vi "Gif.CreatePictureArray.vi"(1 "gloal color table":u32[](array[numeric]), 2 "GraphicControlExtension":T2, 3 "Logical Screen Description":T1, 5 "Index Array":i32[](array[numeric]), 7 "init":bool, 9 "offset":i32, 11 "error in (no error)":errorcluster, 12 "local color table":u32[](array[numeric]), 13 "ImageDescriptor":T3, 14 "bgcolor":u32) -> (4 "image out":u32[][](array[colorbox]), 10 "offset out":i32, 15 "error out":errorcluster)   [LabVIEW 2019]
uses:
  Gif.ImageDescriptor.ctl
  Gif.GraphicControlExtension.ctl
  Gif.LogicalScreenDescriptior.ctl
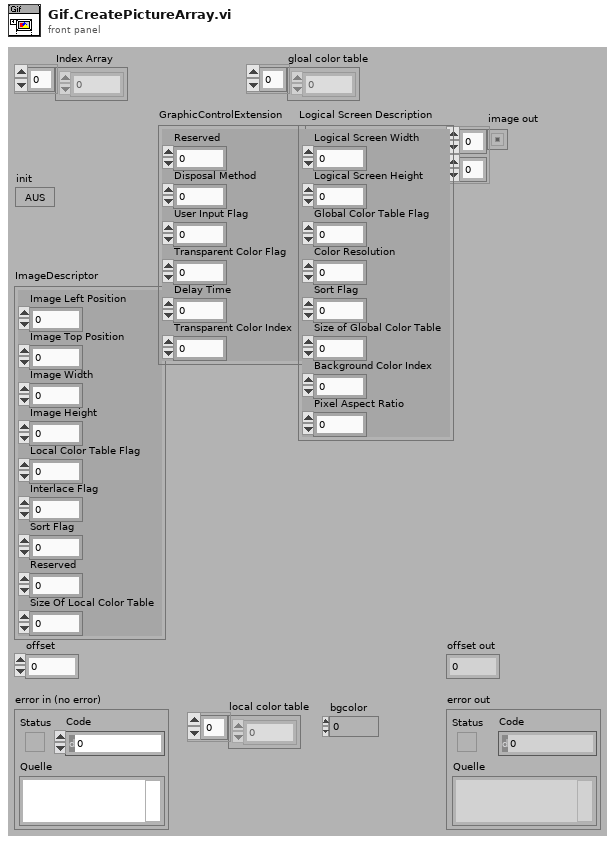
[diagram p1: front panel]
types:
  T1 = typedef "Gif.LogicalScreenDescriptior.ctl" = cluster{"Logical Screen Width":u16, "Logical Screen Height":u16, "Global Color Table Flag":u8, "Color Resolution":u8, "Sort Flag":u8, "Size of Global Color Table":u8, "Background Color Index":u8, "Pixel Aspect Ratio":u8}
  T2 = typedef "Gif.GraphicControlExtension.ctl" = cluster{"Reserved":u8, "Disposal Method":u8, "User Input Flag":u8, "Transparent Color Flag":u8, "Delay Time":u16, "Transparent Color Index":u8}
  T3 = typedef "Gif.ImageDescriptor.ctl" = cluster{"Image Left Position":u16, "Image Top Position":u16, "Image Width":u16, "Image Height":u16, "Local Color Table Flag":u8, "Interlace Flag":u8, "Sort Flag":u8, "Reserved":u8, "Size Of Local Color Table":u8}
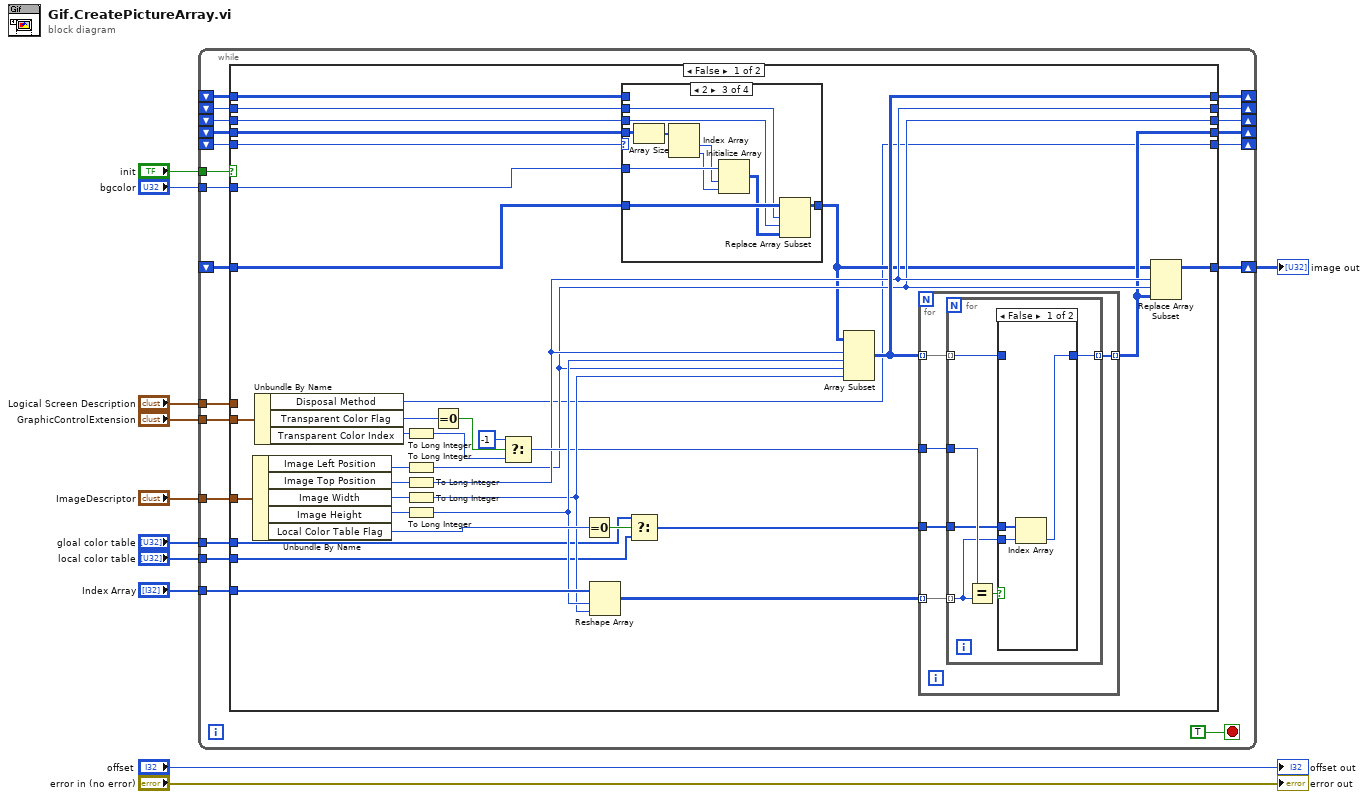
[diagram p0: block diagram]
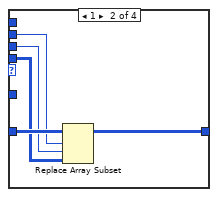
[diagram p3: hidden frame]
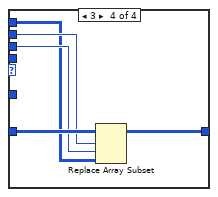
[diagram p4: hidden frame]
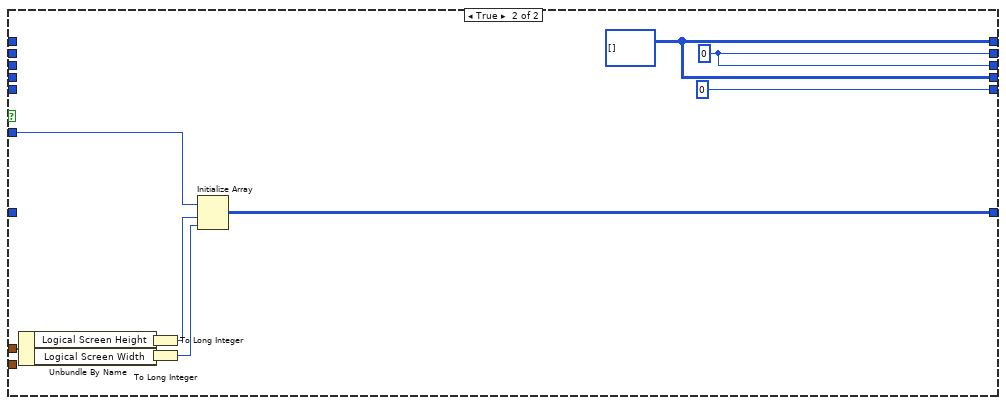
[diagram p6: hidden frame]
diagram:
  n1 = while {
    tunnel: "ImageDescriptor" -> [w32]
    tunnel: "Logical Screen Description" -> [w25]
    tunnel: "GraphicControlExtension" -> [w30]
    tunnel: "Index Array" -> [w28]
    tunnel: "local color table" -> [w27]
    tunnel: "gloal color table" -> [w14]
    shift-right: [w24] -> _
    shift-left: _ -> [w18]
    shift-right: [w23] -> _
    shift-left: _ -> [w17]
    shift-right: [w22] -> _
    shift-left: _ -> [w16]
    shift-right: [w21] -> _
    shift-left: _ -> [w15]
    shift-right: [w20] -> _
    shift-left: _ -> [w19]
    shift-right: [w31] -> w9
    shift-left: _ -> [w29]
    tunnel: "init" -> [w13]
    tunnel: "bgcolor" -> [w12]
    stop <- TRUE stop-if-true
    n2 = case shown="False" w13 {
      tunnel: w32 -> [w67 _]
      tunnel: [w64 w107] -> w31
      tunnel: w30 -> [w59 _]
      tunnel: w29 -> [w33 _]
      tunnel: w28 -> [w57 _]
      tunnel: w27 -> [w54 _]
      tunnel: w25 -> [_ w105]
      tunnel: [w47 w106] -> w24
      tunnel: [w46 w113] -> w23
      tunnel: [w45 w113] -> w22
      tunnel: [w44 w106] -> w21
      tunnel: [w42 u8 0] -> w20
      tunnel: w19 -> [w41 _]
      tunnel: w18 -> [w40 _]
      tunnel: w17 -> [w39 _]
      tunnel: w16 -> [w38 _]
      tunnel: w15 -> [w37 _]
      tunnel: w14 -> [w35 _]
      tunnel: w12 -> [w34 w108]
      frame False {
        n3 = Unbundle By Name(w67) -> ("Image Left Position"=w63:u16, "Image Top Position"=w62:u16, "Image Width"=w60:u16, "Image Height"=w61:u16, "Local Color Table Flag"=w66:u8)
        n4 = Unbundle By Name(w59) -> ("Disposal Method"=w42:u8, "Transparent Color Flag"=w52:u8, "Transparent Color Index"=w58:u8)
        n5 = To Long Integer(number=w58) -> (32bit integer=w50:i32)
        n6 = To Long Integer(number=w63) -> (32bit integer=w45:i32)
        n7 = To Long Integer(number=w62) -> (32bit integer=w46:i32)
        n8 = To Long Integer(number=w60) -> (32bit integer=w55:i32)
        n9 = To Long Integer(number=w61) -> (32bit integer=w56:i32)
        n10 = Equal To 0?(x=w52) -> (x = 0?=w51:bool)
        n11 = Select(t=-1, s=w51, f=w50) -> (s? t:f=w49:i32)
        n12 = Equal To 0?(x=w66) -> (x = 0?=w65:bool)
        n13 = Reshape Array(w57, w56, w55) -> (w53:i32[][])
        n14 = case shown="2" w41 {
          tunnel: w33 -> [w68 w73 w83 w88]
          tunnel: [w68 w72 w82 w87] -> w43
          tunnel: w40 -> [_ _ _ w84]
          tunnel: w39 -> [_ w70 w81 w86]
          tunnel: w38 -> [_ w69 w80 w85]
          tunnel: w37 -> [_ w71 w78 _]
          tunnel: w34 -> [_ _ w79 _]
          frame 0, Default {
          }
          frame 1 {
            n15 = Replace Array Subset(array=w73, new element=w71, index (row)=w70, index (col)=w69) -> (w72:u32[][])
          }
          frame 2 {
            n16 = Array Size(array=w78) -> (size(s)=w77:i32[])
            n17 = Index Array(array=w77) -> (element #1=w76:i32, element #2=w75:i32)  [unwired: 2 in]
            n18 = Initialize Array(w79, w76, w75) -> (w74:u32[][])
            n19 = Replace Array Subset(array=w83, new element=w74, index (row)=w81, index (col)=w80) -> (w82:u32[][])
          }
          frame 3 {
            n20 = Replace Array Subset(array=w88, new element=w84, index (row)=w86, index (col)=w85) -> (w87:u32[][])
          }
        }
        n21 = Select(t=w35, s=w65, f=w54) -> (s? t:f=w36:u32[])
        n22 = Array Subset(array=w43, index (row)=w46, length (row)=w56, index (col)=w45, length (col)=w55) -> (w47:u32[][])
        n23 = for {
          tunnel: w47 -> [w93] mode=indexing
          tunnel: w53 -> [w92] mode=indexing
          tunnel: w36 -> [w91]
          tunnel: w49 -> [w90]
          tunnel: [w89] -> w44 mode=indexing
          n24 = for {
            tunnel: w93 -> [w97] mode=indexing
            tunnel: w92 -> [w94] mode=indexing
            tunnel: w91 -> [w95]
            tunnel: w90 -> [w99]
            tunnel: [w96] -> w89 mode=indexing
            n25 = Equal?(x=w99, y=w94) -> (x = y?=w98:bool)
            n26 = case shown="False" w98 {
              tunnel: w97 -> [_ w103]
              tunnel: [w100 w103] -> w96
              tunnel: w95 -> [w102 _]
              tunnel: w94 -> [w101 _]
              frame False {
                n27 = Index Array(array=w102, index=w101) -> (element=w100:u32)
              }
              frame True {
              }
            }
          }
        }
        n28 = Replace Array Subset(array=w43, new element=w44, index (row)=w46, index (col)=w45) -> (w64:u32[][])
      }
      frame True {
        w113 = 0
        w106 = u32[][] []
        n29 = Unbundle By Name(w105) -> ("Logical Screen Height"=w104:u16, "Logical Screen Width"=w111:u16)
        n30 = To Long Integer(number=w104) -> (32bit integer=w110:i32)
        n31 = To Long Integer(number=w111) -> (32bit integer=w109:i32)
        n32 = Initialize Array(w108, w110, w109) -> (w107:u32[][])
      }
    }
  }
  "image out" <- w9
  "error out" <- "error in (no error)"
  "offset out" <- "offset"
